vi "Save Reference.vi"(9 "Refernce_logical":dbl[](array[numeric]), 10 "Reference path":dbl[][](array[numeric]), 11 "Save Button":bool) -> ()   [LabVIEW 2015]
uses:
  Globals.vi
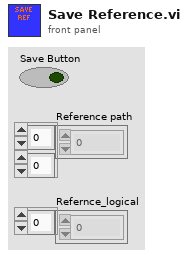
[diagram p1: front panel]
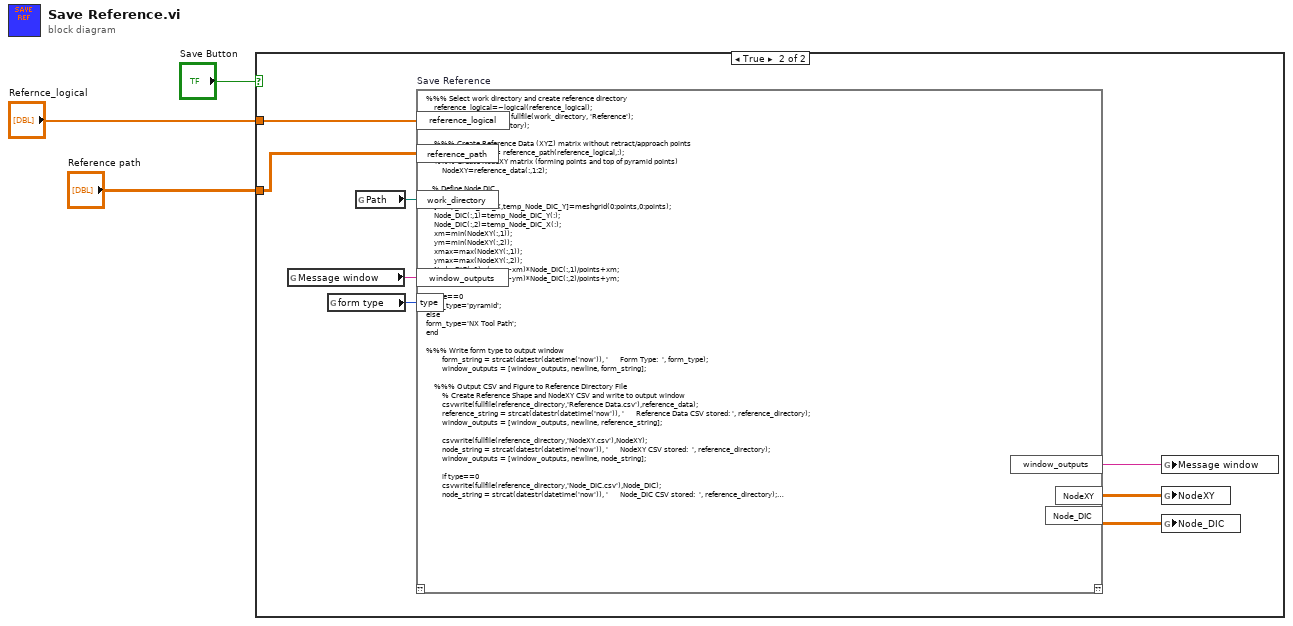
[diagram p0: block diagram]
diagram:
  n1 = case shown="True" "Save Button" {
    tunnel: "Refernce_logical" -> [_ w11]
    tunnel: "Reference path" -> [_ w10]
    frame False {
    }
    frame True {
      n2 = global read "Globals.vi" "Message window"() -> (w8:string)
      n3 = global read "Globals.vi" "form type"() -> (w9:u16)
      n4 = global read "Globals.vi" "Path"() -> (w6:path)
      n5 = script code="%%% Select work directory and create reference directory\n    reference_logical=~logical(reference_logical);\n    reference_directory = fullfile(work_directory, 'Reference');\n    mkdir(reference_directory);\n    \n    %%% Create Reference Data (XYZ) matrix without retract/approach points\n        reference_data = reference_path(reference_logical,:);    \n    %%% Create NodeXY matrix (forming points and top of pyramid points)\n        NodeXY=reference_data(:,1:2);\n     \n   % Define Node DIC \n    points=124;\n    [temp_Node_DIC_X,temp_Node_DIC_Y]=meshgrid(0:points,0:points);\n    Node_DIC(:,1)=temp_Node_DIC_Y(:);\n    Node_DIC(:,2)=temp_Node_DIC_X(:);\n    xm=min(NodeXY(:,1));\n    ym=min(NodeXY(:,2));\n    xmax=max(NodeXY(:,1));\n    ymax=max(NodeXY(:,2));\n    Node_DIC(:,1)=(xmax-xm)*Node_DIC(:,1)/points+xm;\n    Node_DIC(:,2)=(ymax-ym)*Node_DIC(:,2)/points+ym;\n    \nif type==0\nform_type='pyramid';\nelse\nform_type='NX Tool Path';\nend\n\n%%% Write form type to output window \n        form_string = strcat(datestr(datetime('now')), '      Form Type:  ', form_type);\n        window_outputs = [window_outputs, newline, form_string];    \n        \n    %%% Output CSV and Figure to Reference Directory File\n        % Create Reference Shape and NodeXY CSV and write to output window\n        csvwrite(fullfile(reference_directory,'Reference Data.csv'),reference_data);\n        reference_string = strcat(datestr(datetime('now')), '      Reference Data CSV stored: ', reference_directory);\n        window_outputs = [window_outputs, newline, reference_string];\n\n        csvwrite(fullfile(reference_directory,'NodeXY.csv'),NodeXY);\n        node_string = strcat(datestr(datetime('now')), '      NodeXY CSV stored:  ', reference_directory); \n        window_outputs = [window_outputs, newline, node_string];     \n        \n        if type==0\n        csvwrite(fullfile(reference_directory,'Node_DIC.csv'),Node_DIC);\n        node_string = strcat(datestr(datetime('now')), '      Node_DIC CSV stored:  ', reference_directory); \n        window_outputs = [window_outputs, newline, node_string];\n        end\n        \n        % Create Reference Figure    \n        ref_fig = figure;\n        xlabel('X (mm)');\n        ylabel('Y (mm)');\n        zlabel('Z (mm)');\n        plot3(reference_data(:,1),reference_data(:,2),reference_data(:,3));\n        hold on\n        scatter3(reference_data(:,1),reference_data(:,2),reference_data(:,3));\n        hold off\n        savefig(ref_fig, fullfile(reference_directory,'Reference Figure.fig'));\n        reference_fig_string = strcat(datestr(datetime('now')), '      Reference Figure stored:  ', reference_directory);\n        window_outputs = [window_outputs, newline, reference_fig_string];\n  \n    %%% Save inputs to work space\n        fileID = fopen(fullfile(reference_directory,'Reference Pyramid Parameters.txt'),'w');\n        fprintf(fileID,'Reference Pyramid Parameters\\n');\n        fprintf(fileID,'Height (mm): %4.3f\\n',height);\n        fprintf(fileID,'Width (mm): %4.3f\\n',width);\n        fprintf(fileID,'Increment (mm): %4.3f\\n',increment);\n        fprintf(fileID,'Number of Layers: %4.3f\\n',num_layers);\n        fprintf(fileID,'Calculated Depth (mm): %4.3f\\n',(increment*num_layers));\n        fprintf(fileID,'Vertical Angle (degrees): %4.3f\\n',vangle);\n        fprintf(fileID,'Overlap (mm): %4.3f\\n',overlap);\n        fprintf(fileID,'Minimum Point Distance (mm): %4.3f\\n',min_dist);\n        fclose(fileID);\n        referenceinfo_string = strcat(datestr(datetime('now')), '      Reference Information file stored:  ', reference_directory);\n        window_outputs = [window_outputs, newline, referenceinfo_string];\n        \n        % Save reference gridded data\n        x = 0:254;\n        y = 0:254;\n        [X,Y] = meshgrid(x,y);\n        R = scatteredInterpolant(reference_data(:,1),reference_data(:,2),reference_data(:,3));\n        reference_grid = R(X,Y);\n        csvwrite(fullfile(reference_directory, 'Reference Z Gridded Data.csv'),reference_grid);\n        reference_grid_string = strcat(datestr(datetime('now')), '      Reference Gridded .csv stored:  ', reference_directory);\n        window_outputs = [window_outputs, newline, reference_grid_string];\n        \n        % Output line divider\n        window_outputs = [window_outputs, newline, ' ----------- ', newline];" "Save Reference"("reference_logical"=w11, "reference_path"=w10, "type"=w9, "window_outputs"=w8, "work_directory"=w6) -> ("window_outputs"=w7:string, "NodeXY"=w4:dbl[][], "Node_DIC"=w5:dbl[][])  [unwired: 1 in, 1 out]
      n6 = global write "Globals.vi" "Message window"(w7) -> ()
      n7 = global write "Globals.vi" "NodeXY"(w4) -> ()
      n8 = global write "Globals.vi" "Node_DIC"(w5) -> ()
    }
  }
